vi "Initialize.vi"(8 "error in (no error)":errorcluster, 11 "UDP Configuration in":refnum<class "UDP Configurations.lvclass">) -> (0 "error out":errorcluster, 3 "UDP Configuration out":refnum<class "UDP Configurations.lvclass">)   [LabVIEW 2017, in "UDP Configurations.lvclass"]
uses:
  UDP Configurations.lvclass
  C:/Git/DSF/Core/Classes/Component Configuration/Component Configurations.lvclass
  UDP Thread Configuration.lvclass
  C:/Git/DSF/Core/Classes/Configuration/Configuration.lvclass
  Rx Transfer/UDP Transfer Rx Configuration.lvclass
  Tx Transfer/UDP Transfer Tx Configuration.lvclass
  Classes/Component Configuration/Component Configurations.lvclass
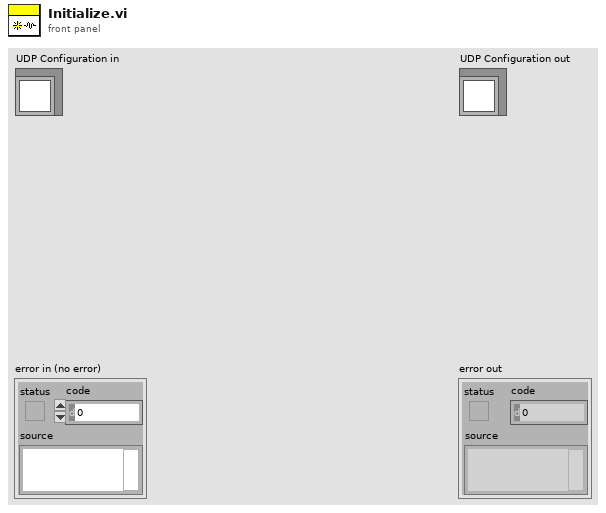
[diagram p1: front panel]
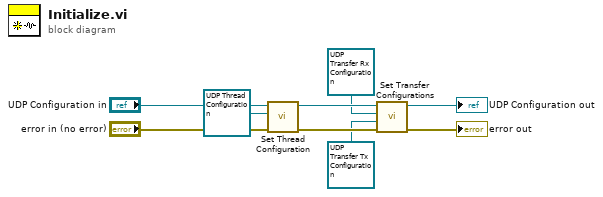
[diagram p0: block diagram]
diagram:
  n1 = call "Set Thread Configuration.vi"("error in (no error)"="error in (no error)", "Thread Configuration"=refnum<class "UDP Thread Configuration.lvclass"> refnum ("DSF Core.lvlib:DSF UDP Thread Configuration"), "Component Configuration in"="UDP Configuration in") -> ("error out"=w6:errorcluster, "Component Configuration out"=w5:refnum<class "UDP Configurations.lvclass">)  [unwired: 7 in]
  n2 = call "Set Transfer Configurations.vi"("error in (no error)"=w6, "Tx Transfer Configuration"=refnum<class "UDP Transfer Tx Configuration.lvclass"> refnum ("DSF Core.lvlib:UDP Tx Transfer Configuration.lvclass"), "Rx Transfer Configuration"=refnum<class "UDP Transfer Rx Configuration.lvclass"> refnum ("DSF Core.lvlib:UDP Rx Transfer Configuration.lvclass"), "Component Configuration in"=w5) -> ("error out"=→"error out":errorcluster, "Component Configuration out"=→"UDP Configuration out":refnum<class "UDP Configurations.lvclass">)  [unwired: 6 in]
